vi "Get Sigma.vi"(8 "error in":errorcluster, 10 "IV in":sgl[](array[numeric]), 11 "DMA in":refnum<class "DMA.lvclass">) -> (0 "error out":errorcluster, 1 "Finished?":bool, 2 "IV Out":sgl[](array[numeric]), 3 "DMA Out":refnum<class "DMA.lvclass">)   [LabVIEW 2015, in "DMA.lvclass"]
uses:
  DMA.lvclass
  DMA.lvclass/DMA.ctl
  <vilib>/Analysis/baseanly.llb/A x Vector.vi
  <vilib>/Analysis/NI_AALBase.lvlib
panel:
  out "x-y":dbl
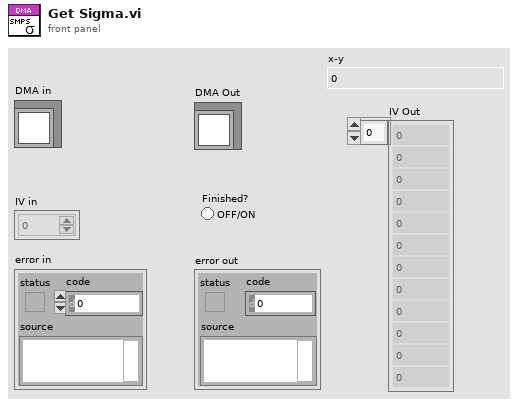
[diagram p1: front panel]
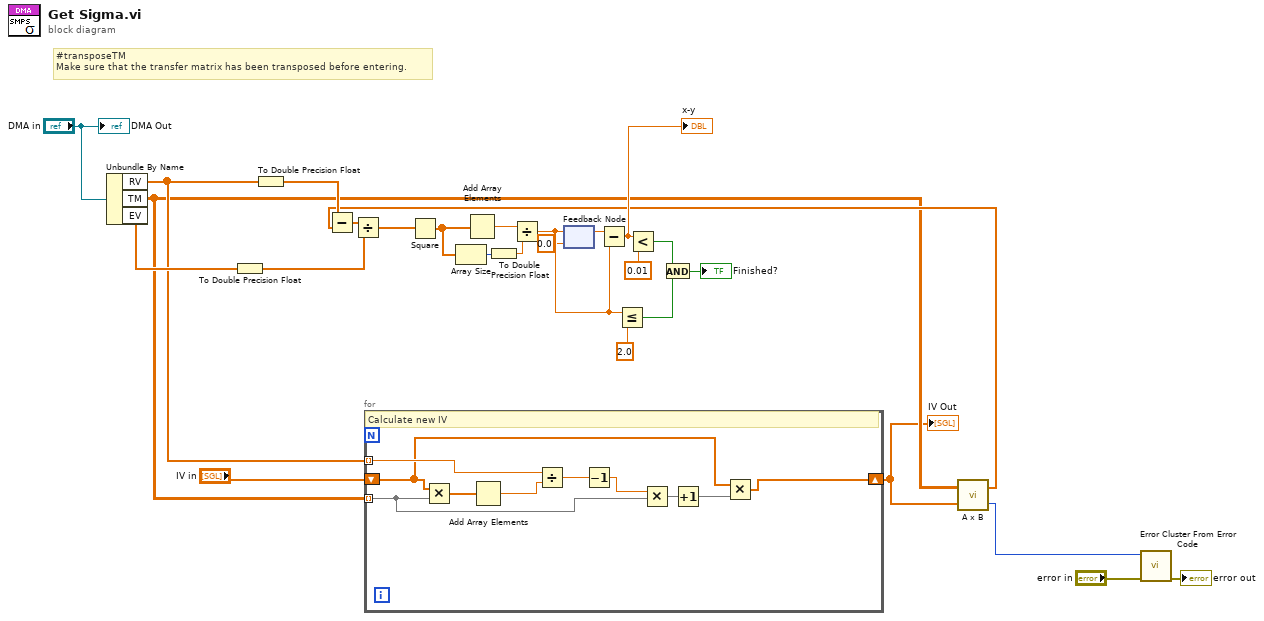
[diagram p0: block diagram]
diagram:
  # "#transposeTM\nMake sure that the transfer matrix has been transposed before entering."
  n1 = Unbundle By Name("DMA in") -> ("RV"=w6:sgl[], "TM"=w2:sgl[][], "EV"=w19:sgl[])
  n2 = To Double Precision Float(number=w19) -> (double precision float=w18:dbl[])
  n3 = To Double Precision Float(number=w6) -> (double precision float=w20:dbl[])
  n4 = for {
    tunnel: w2 -> [w32] mode=indexing
    tunnel: w6 -> [w37] mode=indexing
    shift-right: [w28] -> w1
    shift-left: "IV in" -> [w29]
    # "Calculate new IV"
    n5 = Multiply(x=w29, y=w32) -> (x*y=w36:sgl[])
    n6 = Add Array Elements(numeric array=w36) -> (sum=w35:sgl)
    n7 = Divide(x=w37, y=w35) -> (x/y=w34:sgl)
    n8 = Decrement(x=w34) -> (x-1=w33:sgl)
    n9 = Multiply(x=w33, y=w32) -> (x*y=w31:sgl[])
    n10 = Increment(x=w31) -> (x+1=w30:sgl[])
    n11 = Multiply(x=w29, y=w30) -> (x*y=w28:sgl[])
  }
  "IV Out" <- w1
  n12 = feedback #1(0.0) -> (w15:dbl)
  n13 = call-poly <vilib>:"A x B.vi"("Vector"=w1, "A"=w2) -> ("error"=w4:i32, "A x Vector"=w5:dbl[])
  n14 = Subtract(x=w20, y=w5) -> (x-y=w24:dbl[])
  n15 = Divide(x=w24, y=w18) -> (x/y=w25:dbl[])
  n16 = Square(x=w25) -> (x^2=w26:dbl[])
  n17 = Array Size(array=w26) -> (size(s)=w23:i32)
  n18 = Add Array Elements(numeric array=w26) -> (sum=w27:dbl)
  n19 = To Double Precision Float(number=w23) -> (double precision float=w22:dbl)
  n20 = Divide(x=w27, y=w22) -> (x/y=w14:dbl)
  n21 = feedback-in #1(w14) -> ()
  n22 = Subtract(x=w15, y=w14) -> (x-y=w12:dbl)
  "x-y" <- w12
  n23 = Less Or Equal?(x=w14, y=2.0) -> (x <= y?=w10:bool)
  n24 = Less?(x=w12, y=0.01) -> (x < y?=w9:bool)
  n25 = And(x=w9, y=w10) -> (x .and. y?=→"Finished?":bool)
  n26 = call <vilib>:"Error Cluster From Error Code.vi"("error in (no error)"="error in", "error code (0)"=w4) -> ("error out"=→"error out":errorcluster)  [unwired: 7 in]
  "DMA Out" <- "DMA in"
